vi "histogram_v17.vi"(6 "ROI Descriptor":T2 {"Contours"."Type" items=["No Selection", "Point", "Line", "Rectangle", "Oval", "Polygon", "Freehand Region", "Annulus", "Unused2", "Unused3", "Broken Line", "Freehand Line", "Rotated Rectangle"]}, 8 "useROI":bool, 9 "Color":bool, 11 "Image":T1) -> (0 "error out":errorcluster, 1 "# Sat. Pixels":sgl(slide) scale=0.0..10.0, 2 "mean (ROI)":dbl, 3 "Histograph":T3(graph)={"Starting Value"=-32768.0, "Incremental Value"=1.0, "Histogram"=array[65536 elements]}, 4 "image_size":i32, 5 "max (ROI)":i16, 7 "max_counts":dbl)   [LabVIEW 2017]
uses:
  <vilib>/vision/Image Controls.llb/IMAQ Image.ctl
  <vilib>/vision/NI_Vision_Development_Module.lvlib
panel:
  out "Image Out":T1
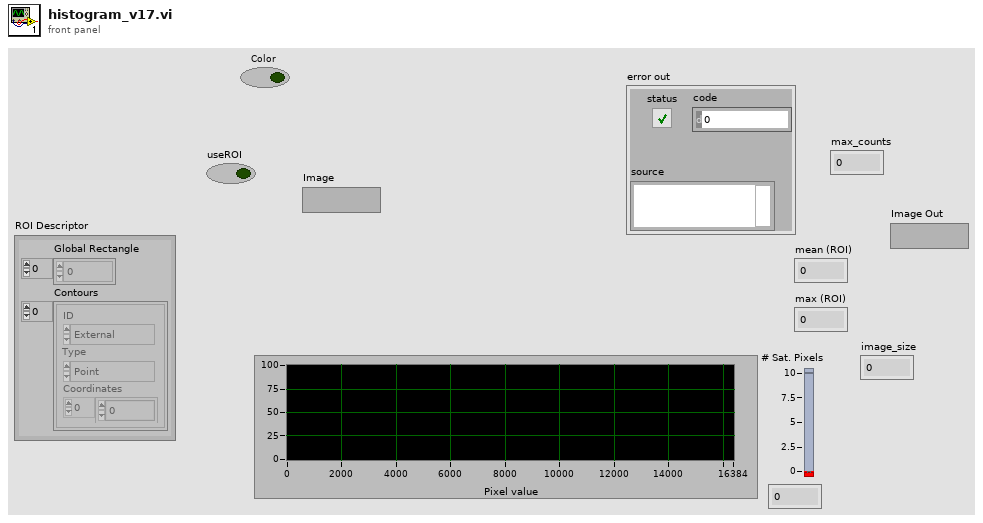
[diagram p1: front panel]
types:
  T1 = typedef "IMAQ Image.ctl" = refnum<image>
  T2 = cluster{"Global Rectangle":i32[], "Contours":cluster{"ID":enum32{"External", "Internal"}, "Type":u32, "Coordinates":i32[]}[]}
  T3 = cluster{"Starting Value":sgl, "Incremental Value":sgl, "Histogram":u32[]}
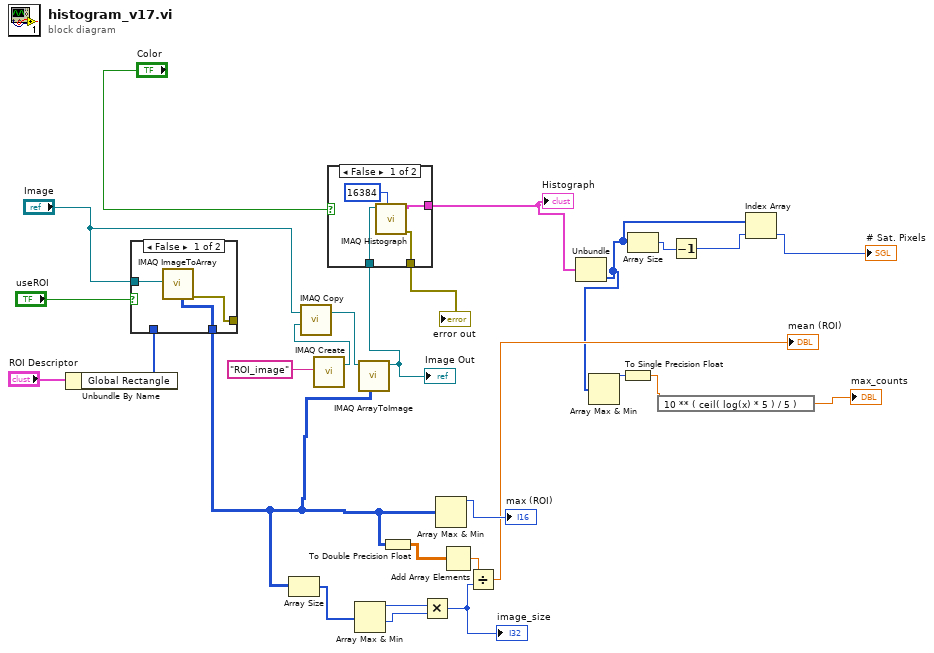
[diagram p0: block diagram]
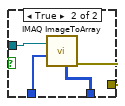
[diagram p2: hidden frame]
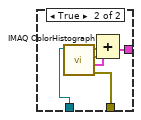
[diagram p3: hidden frame]
diagram:
  n1 = Unbundle By Name("ROI Descriptor") -> ("Global Rectangle"=w21:i32[])
  n2 = case shown="False" "useROI" {
    tunnel: [w29 w32] -> w9
    tunnel: w21 -> [_ w33]
    tunnel: "Image" -> [w30 w34]
    tunnel: [w28 w31] -> _
    frame False {
      n3 = call "IMAQ ImageToArray"("Image"=w30) -> ("Image Pixels (U16)"=w29:u16[][], "error out"=w28:errorcluster)  [unwired: 3 in, 3 out]
    }
    frame True {
      n4 = call "IMAQ ImageToArray"("Optional Rectangle"=w33, "Image"=w34) -> ("Image Pixels (U16)"=w32:u16[][], "error out"=w31:errorcluster)  [unwired: 2 in, 3 out]
    }
  }
  n5 = Array Size(array=w9) -> (size(s)=w15:i32[])
  n6 = call "IMAQ Create"("Image Name"="ROI_image") -> ("New Image"=w6:T1)  [unwired: 4 in, 1 out]
  n7 = call "IMAQ Copy"("Image Dst"=w6, "Image Src"="Image") -> ("Image Dst Out"=w5:T1)  [unwired: 4 in, 1 out]
  n8 = Array Max & Min(array=w15) -> (max value=w14:i32, min value=w10:i32)  [unwired: 2 out]
  n9 = call "IMAQ ArrayToImage"("Image Pixels (U16)"=w9, "Image"=w5) -> ("Image Out"=w8:T1)  [unwired: 8 in, 1 out]
  "Image Out" <- w8
  n10 = case shown="False" "Color" {
    tunnel: [w38 w41] -> w26
    tunnel: [w37 w40] -> w24
    tunnel: w8 -> [w36 w39]
    frame False {
      n11 = call "IMAQ Histograph"("Number of Classes"=16384, "Image"=w36) -> ("error out"=w37:errorcluster, "Histogram Graph"=w38:T3)  [unwired: 6 in, 2 out]
    }
    frame True {
      n12 = call "IMAQ ColorHistograph"("Image Src"=w39) -> ("Red or Hue Histogram Graph"=w44:T3, "Green or Sat Histogram Graph"=w43:T3, "Blue or Luma or Val or Inten Histogram Graph"=w42:T3, "error out"=w40:errorcluster)  [unwired: 5 in]
      n13 = Compound Arithmetic op=ADD(w44, w43, w42) -> (w41:T3)
    }
  }
  "Histograph" <- w26
  "error out" <- w24
  n14 = To Double Precision Float(number=w9) -> (double precision float=w11:dbl[][])
  n15 = Multiply(x=w14, y=w10) -> (x*y=w13:i32)
  "image_size" <- w13
  n16 = Array Max & Min(array=w9) -> (max value=→"max (ROI)":u16)  [unwired: 3 out]
  n17 = Add Array Elements(numeric array=w11) -> (sum=w16:dbl)
  n18 = Divide(x=w16, y=w13) -> (x/y=→"mean (ROI)":dbl)
  n19 = Unbundle(w26) -> ("Histogram"=w4:u32[])  [unwired: 2 out]
  n20 = Array Max & Min(array=w4) -> (max value=w3:u32)  [unwired: 3 out]
  n21 = To Single Precision Float(number=w3) -> (single precision float=w2:sgl)
  n22 = Array Size(array=w4) -> (size(s)=w22:i32)
  n23 = expression code="10 ** ( ceil( log(x) * 5 ) / 5 )"(w2) -> (→"max_counts":sgl)
  n24 = Decrement(x=w22) -> (x-1=w23:i32)
  n25 = Index Array(array=w4, index=w23) -> (element=→"# Sat. Pixels":u32)
